vi "Main RT.vi"() -> ()   [LabVIEW 2015]
uses:
  <vilib>/RioEmbeddedCAN/RioEmbeddedCAN.llb/CANFrameControl.ctl
  Control  rossss.ctl
  PC/QMH Fundamentals - Message Cluster.ctl
  <vilib>/Platform/TimedLoop/XDataNode/timing_clust.ctl
  <vilib>/Platform/TimedLoop/XDataNode/nitl_modes.ctl
  <vilib>/Platform/TimedLoop/XDataNode/wakeup.ctl
  <vilib>/Instr/_visa.llb/VISA Configure Serial Port (Instr).vi
  Global for ROS.vi
  <vilib>/FPGAPlugInAG/sbRIO-9636/niLvFpga_Open_sbRIO-9636.vi
  <vilib>/rvi/interface/common/dynamic/niFpgaDynamicAddResources.vi
  <vilib>/FPGAPlugInAG/Dynamic/niLvFpga_Reset_Dynamic.vi
  <vilib>/FPGAPlugInAG/Dynamic/niLvFpga_Run_Dynamic.vi
  <vilib>/FPGAPlugInAG/Dynamic/niLvFpga_Close_Dynamic.vi
  <vilib>/Platform/TimedLoop/XDataNode/XDataNode.xnode
  <vilib>/rvi/interface/nirviOpenFPGA/nirviOpenFPGA.xnode
  FPGA Bitfiles/Raptorv2_FPGATarget_FPGAMain_QFI8efjbaF8.lvbitx
  FPGA/Main FPGA.vi
  <vilib>/rvi/interface/nirviMethod/nirviMethod.xnode
  <vilib>/rvi/interface/nirviCloseFPGA/nirviCloseFPGA.xnode
  <vilib>/Platform/TimedLoop/XDataNode/XDNodeRunTimeDep.lvlib
  <vilib>/robotics/Protocols/NMEA/NMEA API.lvlib
  <resource>/objmgr/RioEmbeddedCANInterface.rc
  <vilib>/MediaMongrels Ltd/WebSockets/WebSockets/WebSockets.lvlib
panel:
  in  "wej  ID":T1={"STM Lewy ID 1"=2, "STM Prawy ID 2"=1, "IDD 1"=1, "IDD 2"=1}
  in  "send speed over can":T2={"Prêdkosci Prawy"=TRUE, "Prêdkoœci Lewy"=TRUE}
  in  "rosbridge server IP WEBS":string="192.168.1.117"
  in  "rosbridge port WEBS":u16=9090
  out "Return Headers Out":variant
  in  "ros subscribe stop":bool
  out "STEERING out":T3
  in  "STEERING type":T3
  out "Data 2":string
  out "Opcode 2":u8
  out "error out":errorcluster
  in  "Topic to subscribe":string="/STEERING"
  out "GPS Data":T4
  in  "ros send stop":bool
  out "out to ros":T5
  in  "szablon msg velocities":T5
  in  "baud rate":u32=500000
  out "topicSpeed":string
  out "raw JSON frame":string
  out "error out 2":errorcluster
  in  "rosbridge server IP TCP/IP":string="192.168.1.117"
  in  "rosbridge portTCP/IP":u16=9091
  in  "TopicNameSpeed":cluster{"Topic to write":string, "type":string}={"Topic to write"="rio/odom", "type"="sterowanie/velocities"}
  out "output with gps":T6={"op"="publish", "topic"="", "msg"={"layout"={"dim"=[], "data_offset"=0.0}, "data"=[]}}
  out "# elements in queue 2":i32
  in  "error in (no error)":errorcluster
  in  "zero v":T7[](array[typedef])=[{"identifier"=2, "extended?"=FALSE, "type"=0, "payload"=[1, 0, 0, 0, 0, 0, 0]}, {"identifier"=2, "extended?"=FALSE, "type"=0, "payload"=[1]}] {"type" items=["CAN Data", "CAN Remote"]; "identifier" format="%.0x"}
  out "specific error cleared?":bool
  out "# pending insert":i32
  out "# pending remove":i32
  out "# elements in queue":i32
  out "current time":timestamp
  out "Odebrane wiadomoœci z PC":dbl
  out "CAN frame":T7 {"type" items=["CAN Data", "CAN Remote"]; "identifier" format="%.0x"}
  out "wyczyszczona":bool=TRUE
  in  "Wyczyœækolejke":bool
  in  "stop wysylanie":bool
  in  "odczyt CAN-a":bool=TRUE
  out "ilosc mesagy READ CAN":dbl
  in  "Pokaz odczytany CAN":bool=TRUE
  out "CAN Frames":string[][](table) caption="Frames"
  in  "stop odczyt can":bool
  in  "stop zapis can":bool
  out "new data":bool
  in  "odbior udp":bool
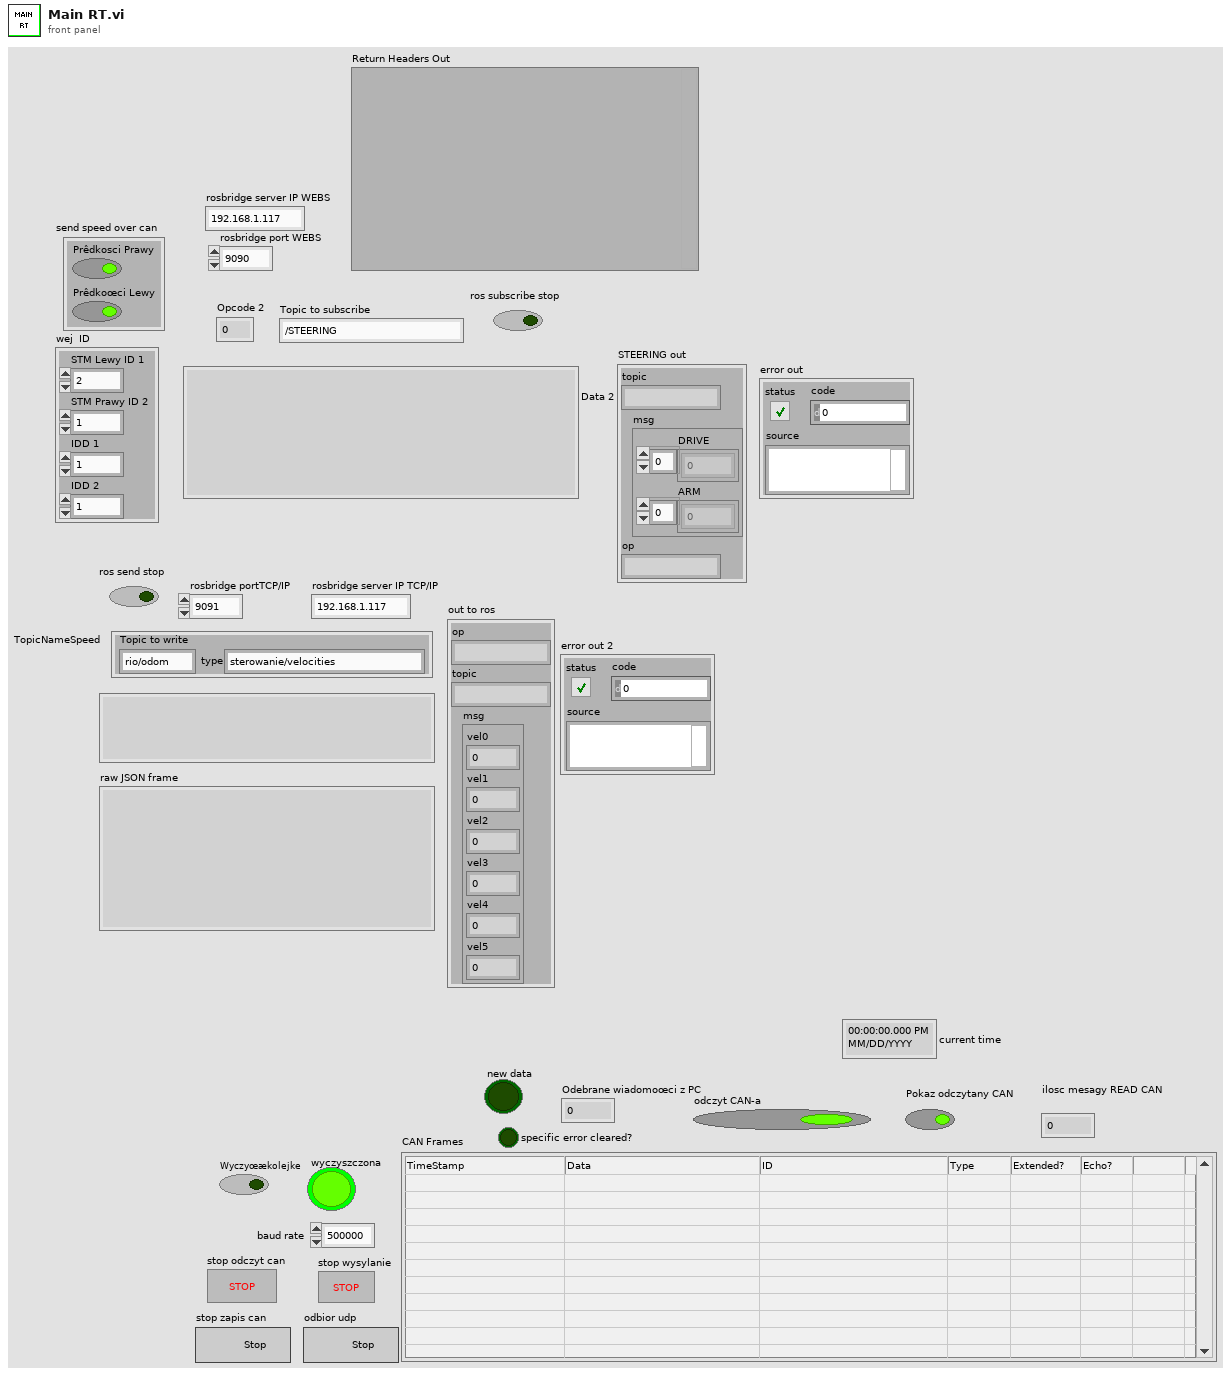
[diagram p1: front panel]
types:
  T1 = cluster{"STM Lewy ID 1":u32, "STM Prawy ID 2":u32, "IDD 1":u8, "IDD 2":u8}
  T2 = cluster{"Prêdkosci Prawy":bool, "Prêdkoœci Lewy":bool}
  T3 = cluster{"topic":string, "msg":cluster{"DRIVE":i16[], "ARM":i8[]}, "op":string}
  T4 = cluster{"oldest read timestamp":timestamp, "latitude":dbl, "longitude":dbl, "speed over ground (knots)":dbl, "true track angle (deg)":dbl, "altitude above mean sea level":dbl, "Fix quality":u16, "Nyumber of satelites":i8}
  T5 = cluster{"op":string, "topic":string, "msg":cluster{"vel0":i16, "vel1":i16, "vel2":i16, "vel3":i16, "vel4":i16, "vel5":i16}}
  T6 = typedef "Control  rossss.ctl" = cluster{"op":string, "topic":string, "msg":cluster{"layout":cluster{"dim":cluster{"stride":i16, "size":i16, "label":string}[], "data_offset":dbl}, "data":i32[]}}
  T7 = typedef "CANFrameControl.ctl" = cluster{"identifier":u32, "extended?":bool, "type":u8, "payload":u8[]}
  T8 = typedef "QMH Fundamentals - Message Cluster.ctl" = cluster{"Message":string, "Message Data":variant}
  T9 = cluster{"Topic to write":string, "TCP Network Connection out":refnum<k5>, "error out":errorcluster}
  T10 = cluster{"DRIVE":refnum<queue>, "KONFIG,PROBE,ARM":refnum<queue>, "ERROR Q":errorcluster, "SEND DATA":refnum<queue>, "TIMEOUT":refnum<queue>, "GIMBALE":refnum<queue>, "SAFETY":refnum<queue>}
  T11 = cluster{"Data":cluster{"date/time string":string, "array of cans":cluster{"identifier":u32, "extended?":bool, "type":u8, "payload":u8[]}[]}, "bool":bool}
  T12 = typedef "XDNodeRunTimeDep.lvlib/timing_clust.ctl" = cluster{"Expected End [f-1]":u64, "Actual End [f-1]":u64, "Finished Late? [f-1]":bool, "Expected End [i-1]":u64, "Actual End [i-1]":u64, "Finished Late? [i-1]":bool, "Expected Start [i]":u64, "Actual Start [i]":u64, "Expected Start [f]":u64, "Actual Start [f]":u64, "Source Name":string, "Structure Name":string, "Period":i64, "Deadline":i64, "Offset":i64, "Start":i64, "Priority":i32, "Timeout":i32, "Mode":T13, "Wakeup Reason":T14, "Error":errorcluster, "Source Type":string, "Secondary Source Type":string, "Global End Time":u64, "Global Start Time":u64, "Frame Duration":u64, "Iteration Duration":u64, "Assigned CPU":i32, "I/O Scan Engine Mode":u32}
  T13 = typedef "XDNodeRunTimeDep.lvlib/nitl_modes.ctl" = enum32{"No Change", "Process missed periods, maintain original phase", "Discard missed periods, maintain original phase", "Process missed periods, ignore original phase", "Discard missed periods, ignore original phase"}
  T14 = typedef "XDNodeRunTimeDep.lvlib/wakeup.ctl" = enum32{"Normal", "Aborted", "Asynchronous wakeup", "Timing source error", "Timed loop error", "Timeout"}
  T15 = cluster{"identifier":u32, "extended?":bool, "type":u8, "payload":u8[]}[]
  T16 = cluster{"identifier":u32, "extended?":bool, "type":u8, "payload":u8[]}
  T17 = cluster{"CAN frame":T7, "GPS Data":cluster{"oldest read timestamp":timestamp, "latitude":dbl, "longitude":dbl, "speed over ground (knots)":dbl, "true track angle (deg)":dbl, "altitude above mean sea level":dbl, "Fix quality":u16, "Nyumber of satelites":i8}}
  T18 = cluster{"Decimal Number":sgl, "Decimal Number":sgl, "Decimal Number":sgl, "Decimal Number":sgl, "Decimal Number":sgl, "Decimal Number":sgl}
  T19 = cluster{"Decimal Number":i16, "Decimal Number":i16, "Decimal Number":i16, "Decimal Number":i16, "Decimal Number":i16, "Decimal Number":i16}
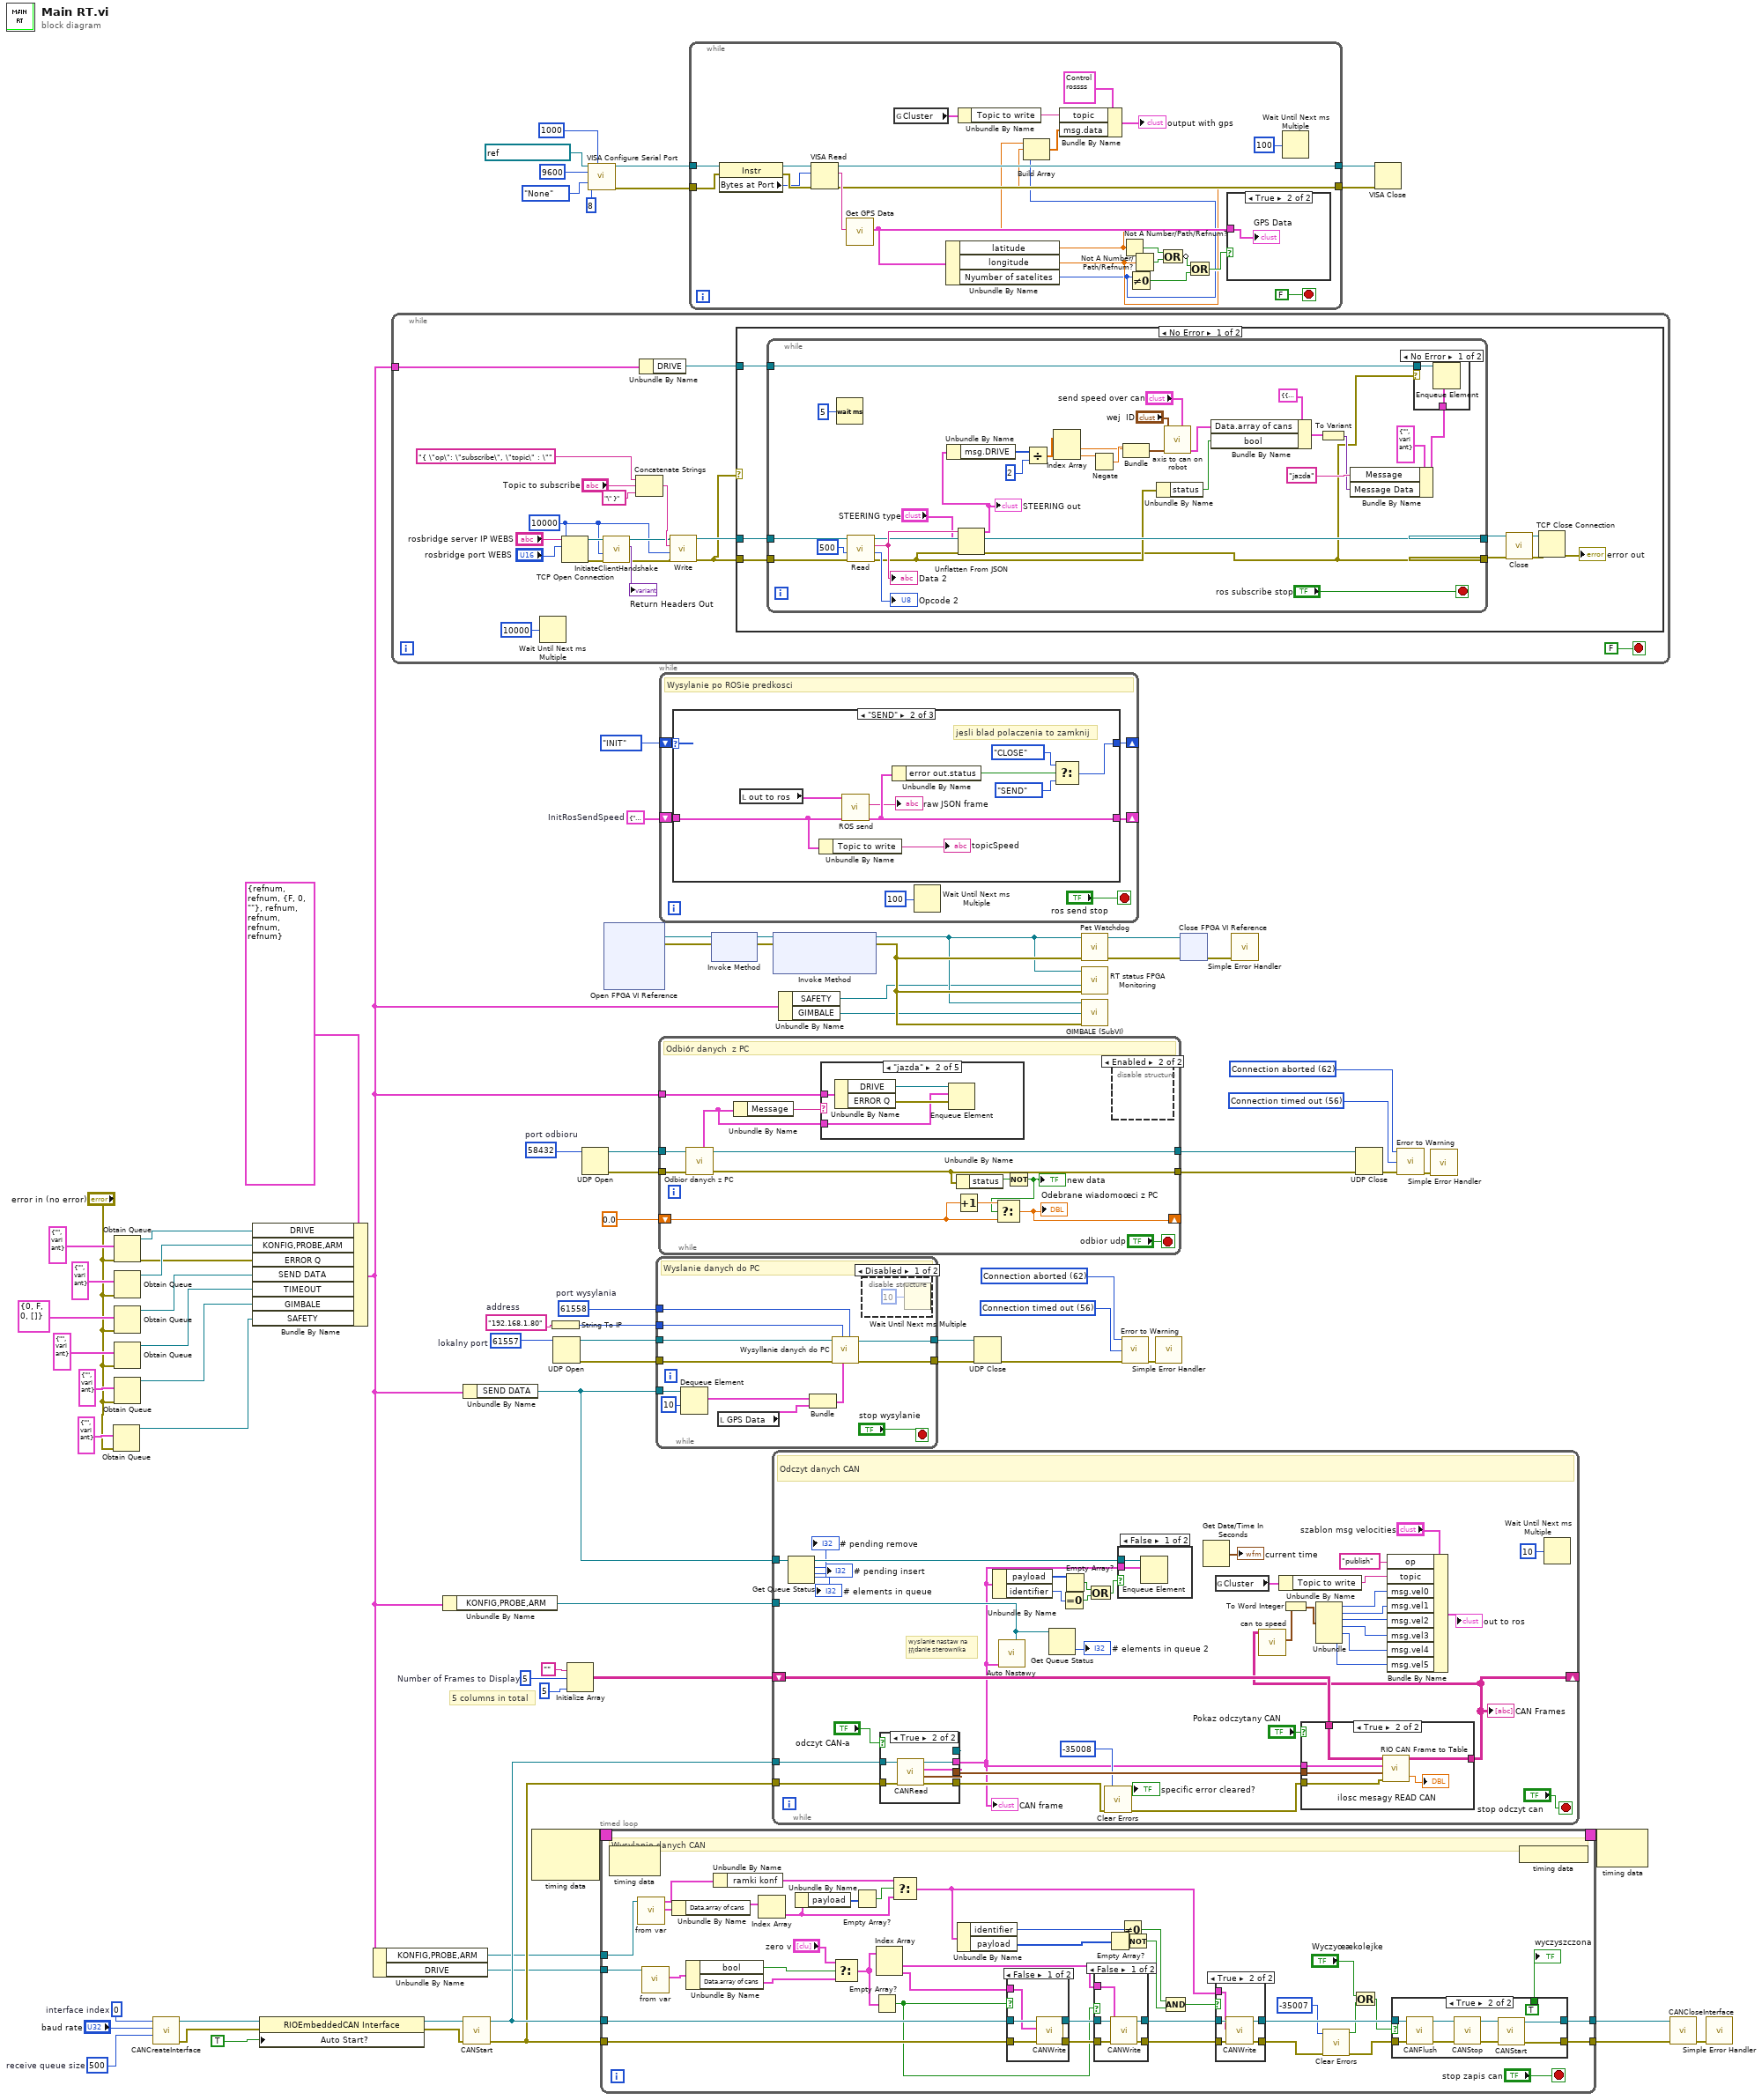
[diagram p0: block diagram]
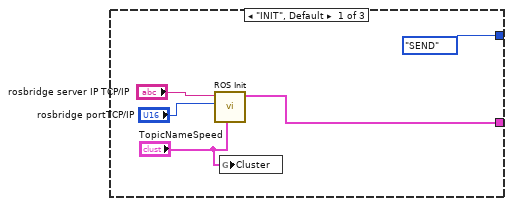
[diagram p4: hidden frame]
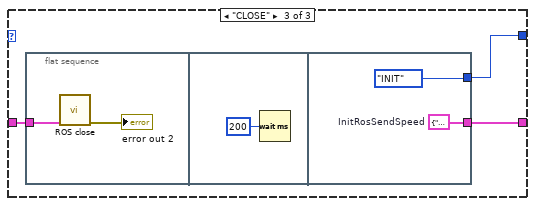
[diagram p5: hidden frame]
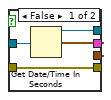
[diagram p9: hidden frame]
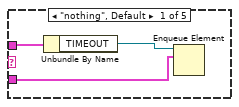
[diagram p11: hidden frame]
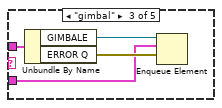
[diagram p12: hidden frame]
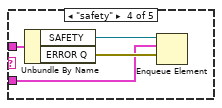
[diagram p13: hidden frame]
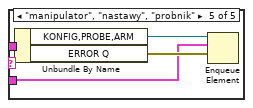
[diagram p14: hidden frame]
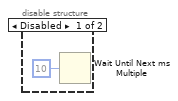
[diagram p15: hidden frame]
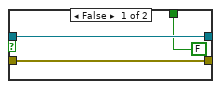
[diagram p16: hidden frame]
diagram:
  w11 = T9 {"Topic to write"="", "TCP Network Connection out"=refnum, "error out"={"status"=FALSE, "code"=0, "source"=""}}  # InitRosSendSpeed
  w79 = u32 500  # receive queue size
  w81 = u32 0  # interface index
  w77 = 5  # Number of Frames to Display
  w43 = u16 58432  # port odbioru
  w47 = 56 items=["No Error", "Argument Error", "Memory Full", "Out of Zone", "End of File", "File Already Open", "Generic File IO Error", "File Not Found", "File Permission Error", "Disk Full", "Duplicate Path", "Too Many Files Open", "Not Enabled", "Resource File Not Found", "Cannot Add Resource", "Resource Not Found", "Image Not Found", "Image Memory Error", "Pen Does Not Exist", "Config Bad Type", "Config Token Not Found", "Config Parse Error", "Config Memory Error", "Bad External Code Format", "Bad External Code Offset", "External Code Not Present", "Null Window", "Destroy Window Mixup", "Null Menu", "Print Aborted", "Bad Print Record", "Print Driver Error", "Windows Error During Print", "Memory Error During Print", "Print Dialog Error", "Generic Print Error", "Invalid Device Refnum", "Device Not Found", "Device Parameter Error", "Device Unit Error", "Can't Open Device", "Device Call Aborted", "Generic Error", "Cancelled By User", "Object ID Too Low", "Object ID Too High", "Object Not In Heap", "Unknown Heap", "Bad DefProc ID", "DefProc Not In Table", "Message Out Of Range", "Null Method", "Unknown Message", "Manager Call Not Supported", "Bad address", "Connection In progress", "Connection timed out", "Connection is already in progress", "Network attribute not supported", "Network error", "Address in use", "System out of memory", "Connection aborted", "Connection refused", "Connection is not connected", "Connection is already connected", "Connection closed", "Initialize error (interapplication manager)", "Bad occurrence", "Wait on unbound occurrence handler", "Occurrence queue overflow", "Bad path", "Semaphore not signaled", "Unrecognized type (interapplication manager)"] ("3rd Error to Convert")
  w46 = 62 items=["No Error", "Argument Error", "Memory Full", "Out of Zone", "End of File", "File Already Open", "Generic File IO Error", "File Not Found", "File Permission Error", "Disk Full", "Duplicate Path", "Too Many Files Open", "Not Enabled", "Resource File Not Found", "Cannot Add Resource", "Resource Not Found", "Image Not Found", "Image Memory Error", "Pen Does Not Exist", "Config Bad Type", "Config Token Not Found", "Config Parse Error", "Config Memory Error", "Bad External Code Format", "Bad External Code Offset", "External Code Not Present", "Null Window", "Destroy Window Mixup", "Null Menu", "Print Aborted", "Bad Print Record", "Print Driver Error", "Windows Error During Print", "Memory Error During Print", "Print Dialog Error", "Generic Print Error", "Invalid Device Refnum", "Device Not Found", "Device Parameter Error", "Device Unit Error", "Can't Open Device", "Device Call Aborted", "Generic Error", "Cancelled By User", "Object ID Too Low", "Object ID Too High", "Object Not In Heap", "Unknown Heap", "Bad DefProc ID", "DefProc Not In Table", "Message Out Of Range", "Null Method", "Unknown Message", "Manager Call Not Supported", "Bad address", "Connection In progress", "Connection timed out", "Connection is already in progress", "Network attribute not supported", "Network error", "Address in use", "System out of memory", "Connection aborted", "Connection refused", "Connection is not connected", "Connection is already connected", "Connection closed", "Initialize error (interapplication manager)", "Bad occurrence", "Wait on unbound occurrence handler", "Occurrence queue overflow", "Bad path", "Semaphore not signaled", "Unrecognized type (interapplication manager)"] ("1st Error to Convert")
  w56 = u16 61557  # lokalny port
  w54 = u16 61558  # port wysylania
  w55 = "192.168.1.80"  # address
  w58 = 56 items=["No Error", "Argument Error", "Memory Full", "Out of Zone", "End of File", "File Already Open", "Generic File IO Error", "File Not Found", "File Permission Error", "Disk Full", "Duplicate Path", "Too Many Files Open", "Not Enabled", "Resource File Not Found", "Cannot Add Resource", "Resource Not Found", "Image Not Found", "Image Memory Error", "Pen Does Not Exist", "Config Bad Type", "Config Token Not Found", "Config Parse Error", "Config Memory Error", "Bad External Code Format", "Bad External Code Offset", "External Code Not Present", "Null Window", "Destroy Window Mixup", "Null Menu", "Print Aborted", "Bad Print Record", "Print Driver Error", "Windows Error During Print", "Memory Error During Print", "Print Dialog Error", "Generic Print Error", "Invalid Device Refnum", "Device Not Found", "Device Parameter Error", "Device Unit Error", "Can't Open Device", "Device Call Aborted", "Generic Error", "Cancelled By User", "Object ID Too Low", "Object ID Too High", "Object Not In Heap", "Unknown Heap", "Bad DefProc ID", "DefProc Not In Table", "Message Out Of Range", "Null Method", "Unknown Message", "Manager Call Not Supported", "Bad address", "Connection In progress", "Connection timed out", "Connection is already in progress", "Network attribute not supported", "Network error", "Address in use", "System out of memory", "Connection aborted", "Connection refused", "Connection is not connected", "Connection is already connected", "Connection closed", "Initialize error (interapplication manager)", "Bad occurrence", "Wait on unbound occurrence handler", "Occurrence queue overflow", "Bad path", "Semaphore not signaled", "Unrecognized type (interapplication manager)"] ("3rd Error to Convert")
  w41 = 62 items=["No Error", "Argument Error", "Memory Full", "Out of Zone", "End of File", "File Already Open", "Generic File IO Error", "File Not Found", "File Permission Error", "Disk Full", "Duplicate Path", "Too Many Files Open", "Not Enabled", "Resource File Not Found", "Cannot Add Resource", "Resource Not Found", "Image Not Found", "Image Memory Error", "Pen Does Not Exist", "Config Bad Type", "Config Token Not Found", "Config Parse Error", "Config Memory Error", "Bad External Code Format", "Bad External Code Offset", "External Code Not Present", "Null Window", "Destroy Window Mixup", "Null Menu", "Print Aborted", "Bad Print Record", "Print Driver Error", "Windows Error During Print", "Memory Error During Print", "Print Dialog Error", "Generic Print Error", "Invalid Device Refnum", "Device Not Found", "Device Parameter Error", "Device Unit Error", "Can't Open Device", "Device Call Aborted", "Generic Error", "Cancelled By User", "Object ID Too Low", "Object ID Too High", "Object Not In Heap", "Unknown Heap", "Bad DefProc ID", "DefProc Not In Table", "Message Out Of Range", "Null Method", "Unknown Message", "Manager Call Not Supported", "Bad address", "Connection In progress", "Connection timed out", "Connection is already in progress", "Network attribute not supported", "Network error", "Address in use", "System out of memory", "Connection aborted", "Connection refused", "Connection is not connected", "Connection is already connected", "Connection closed", "Initialize error (interapplication manager)", "Bad occurrence", "Wait on unbound occurrence handler", "Occurrence queue overflow", "Bad path", "Semaphore not signaled", "Unrecognized type (interapplication manager)"] ("1st Error to Convert")
  # "5 columns in total"
  n1 = Obtain Queue(element data type=T8 {"Message"="", "Message Data"=variant} ("Message Cluster"), error in (no error)="error in (no error)") -> (queue out=w2:refnum<queue>)  [unwired: 3 in, 2 out]
  n2 = Obtain Queue(element data type=T8 {"Message"="", "Message Data"=variant} ("Message Cluster"), error in (no error)="error in (no error)") -> (queue out=w32:refnum<queue>, error out=w30:errorcluster)  [unwired: 3 in, 1 out]
  n3 = Obtain Queue(element data type=T8 {"Message"="", "Message Data"=variant} ("Message Cluster"), error in (no error)="error in (no error)") -> (queue out=w31:refnum<queue>)  [unwired: 3 in, 2 out]
  n4 = Obtain Queue(element data type=T7 {"identifier"=0, "extended?"=FALSE, "type"=0, "payload"=[]} ("CAN frame"), error in (no error)="error in (no error)") -> (queue out=w28:refnum<queue>)  [unwired: 3 in, 2 out]
  n5 = Obtain Queue(element data type=T8 {"Message"="", "Message Data"=variant} ("Message Cluster"), error in (no error)="error in (no error)") -> (queue out=w22:refnum<queue>)  [unwired: 3 in, 2 out]
  n6 = Obtain Queue(element data type=T8 {"Message"="", "Message Data"=variant} ("Message Cluster"), error in (no error)="error in (no error)") -> (queue out=w7:refnum<queue>)  [unwired: 3 in, 2 out]
  n7 = call <vilib>:"CANCreateInterface.vi"("receive queue size (5)"=w79, "baud rate (125000 bps)"="baud rate", "interface index"=w81) -> ("error out"=w37:errorcluster, "interface object out"=w40:refnum<k20>)  [unwired: 7 in]
  n8 = Bundle By Name(cluster=T10 {"DRIVE"=refnum, "KONFIG,PROBE,ARM"=refnum, "ERROR Q"={"status"=FALSE, "code"=0, "source"=""}, "SEND DATA"=refnum, "TIMEOUT"=refnum, "GIMBALE"=refnum, "SAFETY"=refnum}, "DRIVE"=w32, "KONFIG,PROBE,ARM"=w31, "ERROR Q"=w30, "SEND DATA"=w28, "TIMEOUT"=w22, "GIMBALE"=w7, "SAFETY"=w2) -> (w1:T10)
  n9 = property class="RIOEmbeddedCAN Interface"(reference=w40, error in=w37, "Auto Start?"=TRUE) -> (reference out=w38:refnum<k20>, error out=w36:errorcluster)
  n10 = Unbundle By Name(w1) -> ("KONFIG,PROBE,ARM"=w25:refnum<queue>, "DRIVE"=w26:refnum<queue>)
  n11 = while {
    tunnel: w1 -> [w101]
    stop <- FALSE stop-if-true
    w87 = 10000 ("timeout ms (60000)")
    n12 = Wait Until Next ms Multiple(millisecond multiple=u32 10000) -> ()  [unwired: 1 out]
    n13 = TCP Open Connection(address="rosbridge server IP WEBS", remote port or service name="rosbridge port WEBS", timeout ms (60000)=w87) -> (connection ID=w91:refnum<k5>, error out=w90:errorcluster)  [unwired: 2 in]
    n14 = call <vilib>:"InitiateClientHandshake.vi"("error in (no error)"=w90, "timeout ms (5000)"=w87, "WebSocket Connection in"=w91) -> ("error out"=w88:errorcluster, "Return Headers Out"=→"Return Headers Out":variant, "WebSocket Connection out"=w89:refnum<k5>)  [unwired: 6 in]
    n15 = Concatenate Strings("{ \"op\": \"subscribe\", \"topic\" : \"", "Topic to subscribe", "\" }") -> (w98:string)
    n16 = Unbundle By Name(w101) -> ("DRIVE"=w95:refnum<queue>)
    n17 = call <vilib>:"Write.vi"("error in (no error)"=w88, "timeout ms (5000)"=w87, "Data"=w98, "WebSocket Connection in"=w89) -> ("error out"=w84:errorcluster, "WebSocket Connection out"=w96:refnum<k5>)  [unwired: 6 in]
    n18 = case shown="No Error" w84 {
      tunnel: w96 -> [w109 _]
      tunnel: w95 -> [w108 _]
      tunnel: w84 -> [w107 _]
      frame No Error {
        n19 = while {
          tunnel: [w134] -> w104
          tunnel: [w110] -> w105
          tunnel: w109 -> [w139]
          tunnel: w107 -> [w138]
          tunnel: w108 -> [w122]
          stop <- "ros subscribe stop" stop-if-true
          n20 = Wait (ms)(milliseconds to wait=u32 5) -> ()  [unwired: 1 out]
          n21 = call <vilib>:"Read.vi"("error in (no error)"=w138, "timeout ms (5000)"=500, "WebSocket Connection in"=w139) -> ("error out"=w124:errorcluster, "Opcode"=→"Opcode 2":u8, "Data"=w135:string, "WebSocket Connection out"=w134:refnum<k5>)  [unwired: 5 in]
          "Data 2" <- w135
          n22 = Unflatten From JSON(JSON string=w135, type and defaults="STEERING type", error in (no error)=w124) -> (value=w126:T3, error out=w110:errorcluster)  [unwired: 4 in]
          "STEERING out" <- w126
          n23 = Unbundle By Name(w126) -> ("msg.DRIVE"=w130:i16[])
          n24 = Divide(x=w130, y=i16 2) -> (x/y=w132:dbl[])
          n25 = Index Array(array=w132) -> (element #1=w127:dbl, element #2=w129:dbl)  [unwired: 2 in]
          n26 = Negate(x=w129) -> (-x=w128:dbl)
          n27 = Bundle(w128, w127) -> (w114:cluster{dbl, dbl})  [unwired: 1 in]
          n28 = Unbundle By Name(w124) -> ("status"=w123:bool)
          n29 = call "axis to can on robot.vi"("send speed over can"="send speed over can", "wej ster"=w114, "wej  ID"="wej  ID") -> ("array of cans"=w115:T7[])  [unwired: 5 in, 3 out]
          n30 = Bundle By Name(cluster=T11 {"Data"={"date/time string"="", "array of cans"=[]}, "bool"=TRUE} ("jazda"), "Data.array of cans"=w115, "bool"=w123) -> (w125:T11)
          n31 = To Variant(anything=w125) -> (Variant=w118:variant)
          n32 = Bundle By Name(cluster=T8 {"Message"="", "Message Data"=variant} ("Message Cluster"), "Message"="jazda", "Message Data"=w118) -> (w117:T8)
          n33 = case shown="No Error" w110 {
            tunnel: w122 -> [w141 _]
            tunnel: w117 -> [w140 _]
            frame No Error {
              n34 = Enqueue Element(queue=w141, element=w140) -> ()  [unwired: 2 in, 3 out]
            }
            frame Error {
            }
          }
        }
        n35 = call <vilib>:"Close.vi"("error in (no error)"=w105, "WebSocket Connection in"=w104) -> ("error out"=w103:errorcluster, "WebSocket Connection in"=w102:refnum<k5>)  [unwired: 8 in]
        n36 = TCP Close Connection(connection ID=w102, error in (no error)=w103) -> (error out=→"error out":errorcluster)  [unwired: 1 in, 1 out]
      }
      frame Error {
      }
    }
  }
  n37 = Unbundle By Name(w1) -> ("KONFIG,PROBE,ARM"=w24:refnum<queue>)
  n38 = Unbundle By Name(w1) -> ("SEND DATA"=w27:refnum<queue>)
  n39 = call <vilib>:"CANStart.vi"("error in (no error)"=w36, "interface object in"=w38) -> ("error out"=w70:errorcluster, "interface object out"=w71:refnum<k20>)  [unwired: 8 in]
  n40 = node-c288() -> (w83:T12)  [unwired: 2 in]
  n41 = String To IP(1:w55) -> (0:w53:u32)
  n42 = UDP Open(11:w56) -> (port=w52:refnum<k16>, 0:w51:errorcluster)  [unwired: 4 in, 1 out]
  n43 = Initialize Array("" ("Empty String Constant"), w77, 5 ("dimension size")) -> (w72:string[][])
  n44 = UDP Open(11:w43) -> (port=w60:refnum<k16>, 0:w61:errorcluster)  [unwired: 4 in, 1 out]
  n45 = call-poly "VISA Configure Serial Port"("VISA resource name"=refnum<visa-resource-name> "ASRL1::INSTR", "timeout (10sec)"=u32 1000, "baud rate (9600)"=u32 9600, "data bits (8)"=u16 8, "parity (0:none)"=enum16{"None", "Odd", "Even", "Mark", "Space"}."None") -> ("VISA resource name out"=w14:refnum<visa-resource-name>, "error out"=w13:errorcluster)  [unwired: 9 in]
  n46 = timed-loop "Timed Loop" {
    tunnel: w71 -> [w169]
    tunnel: w70 -> [w168]
    tunnel: [w167] -> w74
    tunnel: [w166] -> w73
    timing: w83 -> [_]
    timing-out: [_] -> w82
    tunnel: w26 -> [w152]
    tunnel: w25 -> [w151]
    stop <- "stop zapis can" stop-if-true
    # "Wysylanie danych CAN"
    n47 = node-c288() -> ()  [unwired: 1 in, 1 out]
    n48 = call "from var.vi"("Queue in"=w151) -> ("data jazda"=w149:T11, "data konfig"=w150:cluster{"bool":bool, "ramki konf":T7})  [unwired: 9 in]
    n49 = call "from var.vi"("Queue in"=w152) -> ("data jazda"=w154:T11)  [unwired: 9 in, 1 out]
    n50 = Unbundle By Name(w149) -> ("Data.array of cans"=w148:T15)
    n51 = Unbundle By Name(w154) -> ("bool"=w153:bool, "Data.array of cans"=w142:T15)
    n52 = Unbundle By Name(w150) -> ("ramki konf"=w145:T7)
    n53 = Index Array(array=w148) -> (element=w143:T16)  [unwired: 1 in]
    n54 = Unbundle By Name(w143) -> ("payload"=w147:u8[])
    n55 = Select(t="zero v", s=w153, f=w142) -> (s? t:f=w156:T7[])
    n56 = Empty Array?(array=w147) -> (empty?=w146:bool)
    n57 = Empty Array?(array=w156) -> (empty?=w157:bool)
    n58 = Index Array(array=w156) -> (element #1=w180:T7, element #2=w179:T7)  [unwired: 2 in]
    n59 = Select(t=w145, s=w146, f=w143) -> (s? t:f=w144:T7)
    n60 = Unbundle By Name(w144) -> ("identifier"=w175:u32, "payload"=w176:u8[])
    n61 = case shown="False" w157 {
      tunnel: w169 -> [w215 w216]
      tunnel: w168 -> [w214 w217]
      tunnel: [w213 w216] -> w181
      tunnel: [w212 w217] -> w182
      tunnel: w179 -> [w211 _]
      frame False {
        n62 = call <vilib>:"CANWrite.vi"("error in (no error)"=w214, "CAN frame"=w211, "interface object in"=w215) -> ("error out"=w212:errorcluster, "interface object out"=w213:refnum<k20>)  [unwired: 7 in]
      }
      frame True {
      }
    }
    n63 = case shown="False" w157 {
      tunnel: w182 -> [w208 w210]
      tunnel: [w206 w209] -> w178
      tunnel: [w205 w210] -> w177
      tunnel: w181 -> [w207 w209]
      tunnel: w180 -> [w204 _]
      frame False {
        n64 = call <vilib>:"CANWrite.vi"("error in (no error)"=w208, "CAN frame"=w204, "interface object in"=w207) -> ("error out"=w205:errorcluster, "interface object out"=w206:refnum<k20>)  [unwired: 7 in]
      }
      frame True {
      }
    }
    n65 = Empty Array?(array=w176) -> (empty?=w172:bool)
    n66 = Not Equal To 0?(x=w175) -> (x != 0?=w173:bool)
    n67 = Not(x=w172) -> (.not. x?=w171:bool)
    n68 = Compound Arithmetic op=AND(w173, w171) -> (w174:bool)
    n69 = case shown="True" w174 {
      tunnel: w177 -> [w196 w201]
      tunnel: [w195 w199] -> w165
      tunnel: [w196 w198] -> w170
      tunnel: w178 -> [w195 w200]
      tunnel: w144 -> [_ w197]
      frame False {
      }
      frame True {
        n70 = call <vilib>:"CANWrite.vi"("error in (no error)"=w201, "CAN frame"=w197, "interface object in"=w200) -> ("error out"=w198:errorcluster, "interface object out"=w199:refnum<k20>)  [unwired: 7 in]
      }
    }
    n71 = call <vilib>:"Clear Errors.vi"("error in (no error)"=w170, "specific error code to clear (0: all)"=-35007) -> ("error out"=w162:errorcluster, "specific error cleared?"=w160:bool)  [unwired: 4 in]
    n72 = Or(x="Wyczyœækolejke", y=w160) -> (x .or. y?=w161:bool)
    n73 = case shown="True" w161 {
      tunnel: [w185 w187] -> w167
      tunnel: [w184 w186] -> w166
      tunnel: w165 -> [w185 w194]
      tunnel: w162 -> [w184 w193]
      tunnel: [FALSE TRUE] -> w158
      frame False {
      }
      frame True {
        n74 = call <vilib>:"CANFlush.vi"("error in (no error)"=w193, "interface object in"=w194) -> ("error out"=w190:errorcluster, "interface object out"=w191:refnum<k20>)  [unwired: 8 in]
        n75 = call <vilib>:"CANStop.vi"("error in (no error)"=w190, "interface object in"=w191) -> ("error out"=w189:errorcluster, "interface object out"=w188:refnum<k20>)  [unwired: 8 in]
        n76 = call <vilib>:"CANStart.vi"("error in (no error)"=w189, "interface object in"=w188) -> ("error out"=w186:errorcluster, "interface object out"=w187:refnum<k20>)  [unwired: 8 in]
      }
    }
    "wyczyszczona" <- w158
    n77 = node-c288() -> ()  [unwired: 1 out]
  }
  n78 = xnode "Open FPGA VI Reference"() -> ("FPGA VI Reference Out"=w65:refnum<k20>, "error out"=w66:errorcluster)  [unwired: 2 in]
  n79 = while {
    tunnel: w54 -> [w225]
    tunnel: w53 -> [w226]
    tunnel: w52 -> [w229]
    tunnel: w51 -> [w228]
    tunnel: [w224] -> w50
    tunnel: [w223] -> w49
    tunnel: w27 -> [w220]
    stop <- "stop wysylanie" stop-if-true
    # "Wyslanie danych do PC"
    n80 = Dequeue Element(queue=w220, timeout in ms (-1)=10) -> (element=w221:T7)  [unwired: 1 in, 3 out]
    n81 = local read "GPS Data"() -> (w222:T4)
    n82 = Bundle("CAN frame"=w221, "GPS Data"=w222) -> (w218:T17)  [unwired: 1 in]
    n83 = call "Wysyllanie danych do PC .vi"("remote port"=w225, "output cluster 2"=w218, "adres"=w226, "error in (no error)"=w228, "UDP Network Connection in"=w229) -> ("error out"=w223:errorcluster, "UDP Network Connection out"=w224:refnum<k16>)  [unwired: 5 in]
    n84 = disable-structure shown="Disabled" {
      frame Disabled {
        n85 = Wait Until Next ms Multiple(millisecond multiple=u32 10) -> ()  [unwired: 1 out]
      }
      frame Enabled {
      }
    }
  }
  n86 = while {
    tunnel: w60 -> [w240]
    tunnel: w61 -> [w239]
    tunnel: [w242] -> w62
    tunnel: [w243] -> w44
    shift-right: [w236] -> _
    shift-left: 0.0 -> [w235]
    tunnel: w1 -> [w232]
    stop <- "odbior udp" stop-if-true
    # "Odbiór danych  z PC"
    n87 = call "Odbior danych z PC .vi"("error in (no error)"=w239, "connection ID"=w240) -> ("error out"=w242:errorcluster, "connection ID out"=w243:refnum<k16>, "Output Data"=w231:T8)  [unwired: 7 in]
    n88 = Unbundle By Name(w231) -> ("Message"=w233:string)
    n89 = case shown="\"jazda\"" w233 {
      tunnel: w232 -> [w246 w248 w252 w256 w259]
      tunnel: w231 -> [w244 w247 w251 w255 w260]
      frame "nothing", Default {
        n90 = Unbundle By Name(w246) -> ("TIMEOUT"=w245:refnum<queue>)
        n91 = Enqueue Element(queue=w245, element=w244) -> ()  [unwired: 2 in, 3 out]
      }
      frame "jazda" {
        n92 = Unbundle By Name(w248) -> ("DRIVE"=w250:refnum<queue>, "ERROR Q"=w249:errorcluster)
        n93 = Enqueue Element(queue=w250, element=w247, error in (no error)=w249) -> ()  [unwired: 1 in, 3 out]
      }
      frame "gimbal" {
        n94 = Unbundle By Name(w252) -> ("GIMBALE"=w254:refnum<queue>, "ERROR Q"=w253:errorcluster)
        n95 = Enqueue Element(queue=w254, element=w251, error in (no error)=w253) -> ()  [unwired: 1 in, 3 out]
      }
      frame "safety" {
        n96 = Unbundle By Name(w256) -> ("SAFETY"=w258:refnum<queue>, "ERROR Q"=w257:errorcluster)
        n97 = Enqueue Element(queue=w258, element=w255, error in (no error)=w257) -> ()  [unwired: 1 in, 3 out]
      }
      frame "manipulator", "nastawy", "probnik" {
        n98 = Unbundle By Name(w259) -> ("KONFIG,PROBE,ARM"=w262:refnum<queue>, "ERROR Q"=w261:errorcluster)
        n99 = Enqueue Element(queue=w262, element=w260, error in (no error)=w261) -> ()  [unwired: 1 in, 3 out]
      }
    }
    n100 = Increment(x=w235) -> (x+1=w237:dbl)
    n101 = Unbundle By Name(w242) -> ("status"=w238:bool)
    n102 = Not(x=w238) -> (.not. x?=w234:bool)
    "new data" <- w234
    n103 = Select(t=w237, s=w234, f=w235) -> (s? t:f=w236:dbl)
    "Odebrane wiadomoœci z PC" <- w236
    n104 = disable-structure shown="Enabled" {
      frame Disabled {
        n105 = Wait Until Next ms Multiple(millisecond multiple=u32 10) -> ()  [unwired: 1 out]
      }
      frame Enabled {
      }
    }
  }
  n106 = while {
    shift-right: [w267] -> _
    shift-left: w11 -> [w266]
    shift-right: [w265] -> _
    shift-left: enum16{"INIT", "CLOSE", "SEND"}."INIT" -> [w269]
    stop <- "ros send stop" stop-if-true
    # "Wysylanie po ROSie predkosci"
    n107 = case shown="\"SEND\"" w269 {
      tunnel: [w272 w280 w284] -> w267
      tunnel: w266 -> [_ w277 w286]
      tunnel: [enum16{"INIT", "CLOSE", "SEND"}."SEND" w283 w285] -> w265
      frame "INIT", Default {
        n108 = call "ROS Init.vi"("topic"="TopicNameSpeed", "rosbridge port"="rosbridge portTCP/IP", "rosbridge  IP"="rosbridge server IP TCP/IP") -> ("output"=w272:T9)  [unwired: 7 in, 1 out]
        n109 = global write "Global for ROS.vi" "Cluster"("TopicNameSpeed") -> ()
      }
      frame "SEND" {
        # "jesli blad polaczenia to zamknij"
        n110 = local read "out to ros"() -> (w275:T5)
        n111 = Unbundle By Name(w277) -> ("Topic to write"=→"topicSpeed":string)
        n112 = call "ROS send.vi"("ConnectionIn"=w277, "dataIn"=w275) -> ("ConnectioOut"=w280:T9, "rawJSONOut"=→"raw JSON frame":string)  [unwired: 8 in]
        n113 = Unbundle By Name(w280) -> ("error out.status"=w279:bool)
        n114 = Select(t=enum16{"INIT", "CLOSE", "SEND"}."CLOSE", s=w279, f=enum16{"INIT", "CLOSE", "SEND"}."SEND") -> (s? t:f=w283:enum16{"INIT", "CLOSE", "SEND"})
      }
      frame "CLOSE" {
        n115 = flat-sequence {
          tunnel: w286 -> [w287]
          tunnel: [enum16{"INIT", "CLOSE", "SEND"}."INIT"] -> w285
          tunnel: [w290] -> w284
          frame #0 {
            n116 = call "ROS close.vi"("DataIn"=w287) -> ("error out"=→"error out 2":errorcluster)  [unwired: 8 in, 2 out]
          }
          frame #1 {
            n117 = Wait (ms)(milliseconds to wait=u32 200) -> ()  [unwired: 1 out]
          }
          frame #2 {
            w290 = T9 {"Topic to write"="", "TCP Network Connection out"=refnum, "error out"={"status"=FALSE, "code"=0, "source"=""}}  # InitRosSendSpeed
          }
        }
      }
    }
    n118 = Wait Until Next ms Multiple(millisecond multiple=u32 100 ("milliseconds to wait")) -> ()  [unwired: 1 out]
  }
  n119 = while {
    tunnel: [w309] -> w21
    tunnel: [w308] -> w20
    tunnel: w14 -> [w307]
    tunnel: w13 -> [w306]
    stop <- FALSE stop-if-true
    n120 = property class="Instr"(reference=w307, error in=w306) -> (reference out=w314:refnum<visa-resource-name>, error out=w313:errorcluster, "Bytes at Port"=w311:u32)
    n121 = VISA Read(VISA resource name=w314, byte count=w311, error in (no error)=w313) -> (VISA resource name out=w309:refnum<visa-resource-name>, read buffer=w312:string, error out=w308:errorcluster)  [unwired: 1 out]
    n122 = call <vilib>:"Get GPS Data.vi"("sensor data"=w312) -> ("GPS Data"=w305:T4)  [unwired: 8 in, 2 out]
    n123 = global read "Global for ROS.vi" "Cluster"() -> (w292:cluster{"Topic to write":string, "type":string})
    n124 = Unbundle By Name(w305) -> ("latitude"=w295:dbl, "longitude"=w294:dbl, "Nyumber of satelites"=w293:i8)
    n125 = Unbundle By Name(w292) -> ("Topic to write"=w297:string)
    n126 = Build Array(w295, w294, w293) -> (w296:dbl[])
    n127 = Bundle By Name(cluster=T6 {"op"="publish", "topic"="rio", "msg"={"layout"={"dim"=[{"stride"=0, "size"=0, "label"="a"}], "data_offset"=0.0}, "data"=[1, 0, 0, 0, 0, 0, 0]}} ("output cluster"), "topic"=w297, "msg.data"=w296) -> (→"output with gps":T6)
    n128 = Not A Number/Path/Refnum?(number/path/refnum=w295) -> (NaN/Path/Refnum?=w303:bool)
    n129 = Not Equal To 0?(x=w293) -> (x != 0?=w300:bool)
    n130 = Not A Number/Path/Refnum?(number/path/refnum=w294) -> (NaN/Path/Refnum?=w304:bool)
    n131 = Compound Arithmetic op=OR(w303, w304) -> (invert w302:bool)
    n132 = Or(x=w302, y=w300) -> (x .or. y?=w301:bool)
    n133 = case shown="True" w301 {
      tunnel: w305 -> [_ w316]
      frame False {
      }
      frame True {
        "GPS Data" <- w316
      }
    }
    n134 = Wait Until Next ms Multiple(millisecond multiple=u32 100) -> ()  [unwired: 1 out]
  }
  n135 = xnode "Invoke Method"("FPGA VI Reference In"=w65, "error in"=w66) -> ("FPGA VI Reference Out"=w67:refnum<k20>, "error out"=w68:errorcluster)
  n136 = while "Timed Loop" {
    shift-right: [w330] -> _
    shift-left: w72 -> [w354]
    tunnel: w71 -> [w356]
    tunnel: w70 -> [w355]
    tunnel: w27 -> [w339]
    tunnel: w24 -> [w337]
    stop <- "stop odczyt can" stop-if-true
    # "wyslanie nastaw na \n抗danie sterownika"
    # "Odczyt danych CAN"
    n137 = Get Queue Status(queue=w339) -> (queue out=w349:refnum<queue>, # pending remove=→"# pending remove":i32, # pending insert=→"# pending insert":i32, # elements in queue=→"# elements in queue":i32)  [unwired: 2 in, 4 out]
    n138 = case shown="True" "odczyt CAN-a" {
      tunnel: w356 -> [w367 w374]
      tunnel: w355 -> [w368 w373]
      tunnel: [w366 w372] -> w352
      tunnel: [w368 w371] -> w343
      tunnel: [_ w369] -> w336
      tunnel: [w367 w370] -> _
      frame False {
        n139 = Get Date/Time In Seconds() -> (seconds since 1Jan1904=w366:timestamp)
      }
      frame True {
        n140 = call <vilib>:"CANRead.vi"("error in (no error)"=w373, "interface object in"=w374) -> ("error out"=w371:errorcluster, "timestamp"=w372:timestamp, "CAN frame"=w369:T7, "interface object out"=w370:refnum<k20>)  [unwired: 6 in]
      }
    }
    "CAN frame" <- w336
    n141 = Unbundle By Name(w336) -> ("payload"=w335:u8[], "identifier"=w334:u32)
    n142 = call "Auto Nastawy.vi"("queue"=w337, "CAN ramki in"=w336) -> ()  [unwired: 10 in]
    n143 = Get Queue Status(queue=w337) -> (# elements in queue=→"# elements in queue 2":i32)  [unwired: 2 in, 7 out]
    n144 = Equal To 0?(x=w334) -> (x = 0?=w331:bool)
    n145 = Empty Array?(array=w335) -> (empty?=w332:bool)
    n146 = Compound Arithmetic op=OR(w332, w331) -> (w333:bool)
    n147 = call <vilib>:"Clear Errors.vi"("error in (no error)"=w343, "specific error code to clear (0: all)"=-35008) -> ("error out"=w342:errorcluster, "specific error cleared?"=→"specific error cleared?":bool)  [unwired: 4 in]
    n148 = case shown="False" w333 {
      tunnel: w349 -> [w358 _]
      tunnel: w336 -> [w357 _]
      frame False {
        n149 = Enqueue Element(queue=w358, element=w357) -> ()  [unwired: 2 in, 3 out]
      }
      frame True {
      }
    }
    n150 = Get Date/Time In Seconds() -> (seconds since 1Jan1904=→"current time":timestamp)
    n151 = global read "Global for ROS.vi" "Cluster"() -> (w328:cluster{"Topic to write":string, "type":string})
    n152 = Unbundle By Name(w328) -> ("Topic to write"=w329:string)
    n153 = case shown="True" "Pokaz odczytany CAN" {
      tunnel: [w359 w365] -> w330
      tunnel: w354 -> [w359 w363]
      tunnel: w352 -> [_ w362]
      tunnel: w336 -> [_ w361]
      tunnel: w342 -> [_ w360]
      frame False {
      }
      frame True {
        n154 = call "RIO CAN Frame to Table.vi"("error in (no error)"=w360, "timestamp"=w362, "CAN frame"=w361, "Old CAN Frames"=w363) -> ("New CAN Frames"=w365:string[][], "Iloœæ wiadomoœci CAN odebranych"=→"ilosc mesagy READ CAN":dbl)  [unwired: 6 in]
      }
    }
    "CAN Frames" <- w330
    n155 = call "can to speed.vi"("Input can Array"=w330) -> ("Napedy"=w317:T18)  [unwired: 8 in, 2 out]
    n156 = To Word Integer(number=w317) -> (16bit integer=w326:T19)
    n157 = Unbundle(w326) -> ("Decimal Number"=w325:i16, "Decimal Number"=w324:i16, "Decimal Number"=w323:i16, "Decimal Number"=w320:i16, "Decimal Number"=w319:i16, "Decimal Number"=w318:i16)
    n158 = Bundle By Name(cluster="szablon msg velocities", "op"="publish", "topic"=w329, "msg.vel0"=w325, "msg.vel1"=w324, "msg.vel2"=w323, "msg.vel3"=w320, "msg.vel4"=w319, "msg.vel5"=w318) -> (→"out to ros":T5)
    n159 = Wait Until Next ms Multiple(millisecond multiple=u32 10) -> ()  [unwired: 1 out]
  }
  n160 = xnode "Invoke Method"("FPGA VI Reference In"=w67, "error in"=w68) -> ("FPGA VI Reference Out"=w9:refnum<k20>, "error out"=w10:errorcluster)  [unwired: 1 in]
  n161 = Unbundle By Name(w1) -> ("SAFETY"=w5:refnum<queue>, "GIMBALE"=w6:refnum<queue>)
  n162 = UDP Close(connection ID=w50, 8:w49) -> (error out=w59:errorcluster)  [unwired: 1 out]
  n163 = call "Pet Watchdog.vi"("ErrorIn"=w10, "FPGA VI Reference In"=w9) -> ("error Out"=w69:errorcluster, "FPGA VI Reference Out"=w63:refnum<k20>)  [unwired: 8 in]
  n164 = call "RT status FPGA Monitoring.vi"("error In"=w10, "SafetyQueue"=w5, "FPGA VI Reference In"=w9) -> ()  [unwired: 9 in]
  n165 = call "GIMBALE (SubVI).vi"("error In"=w10, "GIMBALE Queue"=w6, "Refnum in"=w9) -> ()  [unwired: 9 in]
  n166 = call <vilib>:"Error to Warning.vi"("1st Error to Convert"=w41, "3rd Error to Convert"=w58, "error in"=w59) -> ("warning out"=w57:errorcluster)  [unwired: 3 in, 9 out]
  n167 = call <vilib>:"Simple Error Handler.vi"("error in (no error)"=w57) -> ()  [unwired: 1 in, 8 out]
  n168 = xnode "Close FPGA VI Reference"("FPGA VI Reference In"=w63, "error in"=w69) -> ("error out"=w64:errorcluster)
  n169 = call <vilib>:"Simple Error Handler.vi"("error in (no error)"=w64) -> ()  [unwired: 1 in, 8 out]
  n170 = UDP Close(connection ID=w44, 8:w62) -> (error out=w45:errorcluster)  [unwired: 1 out]
  n171 = VISA Close(VISA resource name=w21, error in (no error)=w20) -> ()  [unwired: 1 out]
  n172 = call <vilib>:"Error to Warning.vi"("1st Error to Convert"=w46, "3rd Error to Convert"=w47, "error in"=w45) -> ("warning out"=w48:errorcluster)  [unwired: 3 in, 9 out]
  n173 = call <vilib>:"Simple Error Handler.vi"("error in (no error)"=w48) -> ()  [unwired: 1 in, 8 out]
  n174 = node-c288(w82) -> ()  [unwired: 1 out]
  n175 = call <vilib>:"CANCloseInterface.vi"("error in (no error)"=w73, "interface object in"=w74) -> ("error out"=w75:errorcluster)  [unwired: 9 in]
  n176 = call <vilib>:"Simple Error Handler.vi"("error in (no error)"=w75) -> ()  [unwired: 4 in, 5 out]
